vi "Proceed.vi"(7 "component is ready (Y)":bool=TRUE, 8 "error in (no error)":errorcluster, 10 "ProceedMessage":refnum<class "ProceedMessage.lvclass">, 11 "ExampleClassC in":refnum<class "ExampleClassC.lvclass">) -> (0 "error out":errorcluster, 2 "all observers are ready?":bool, 3 "ExampleClassC out":refnum<class "ExampleClassC.lvclass">)   [LabVIEW 2012, in "ExampleClassC.lvclass"]
doc: "The Proceed method is used to check if your component is ready. Also it checks if the observers are ready. When the observers and the component are ready, it sends the proceed to its observee. If it's the highest observee, it distributes a stop command."
uses:
  ExampleClassC.lvclass
  <vilib>/Distrio/Murmex/ProceedMessage/ProceedMessage.lvclass
  <vilib>/Distrio/Murmex/Murmex/Murmex.lvclass
panel:
  # "This method is called when the PROCEED\ntrigger is sent. \n\nOverride this method when your component needs to\nrespond to this trigger. \n\nCall parent for proper implementation"
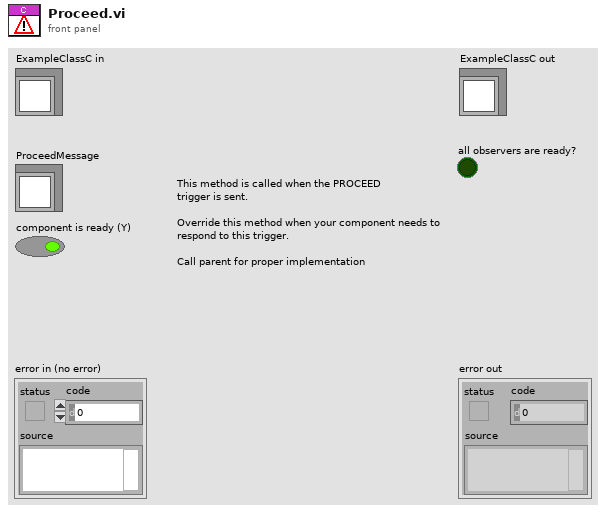
[diagram p1: front panel]
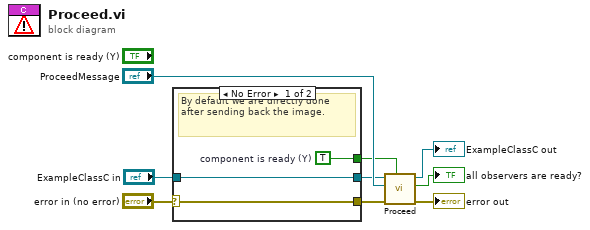
[diagram p0: block diagram]
diagram:
  n1 = case shown="No Error" "error in (no error)" {
    selector: "error in (no error)" -> [w10 w14]
    tunnel: [w12 _] -> w1
    tunnel: [w11 w13] -> w2
    tunnel: "ExampleClassC in" -> [w11 w13]
    tunnel: [w10 w14] -> w4
    frame No Error {
      w12 = TRUE  # component is ready (Y)
      # "By default we are directly done after sending back the image."
    }
    frame Error {
    }
  }
  n2 = call-parent "Proceed.vi"("component is ready (Y)"=w1, "error in (no error)"=w4, "ProceedMessage"="ProceedMessage", "Murmex in"=w2) -> ("error out"=→"error out":errorcluster, "all observers are ready?"=→"all observers are ready?":bool, "Murmex out"=→"ExampleClassC out":refnum<class "ExampleClassC.lvclass">)  [unwired: 5 in]
